vi "Bind Timestamp (Text).vi"(8 "error in (no error)":errorcluster, 10 "Time Stamp":timestamp, 11 "SQL Statement in":refnum<class "SQL Statement.lvclass">) -> (0 "error out":errorcluster, 3 "SQL Statement out":refnum<class "SQL Statement.lvclass">)   [LabVIEW 2011, in "SQLite.lvlib" / "SQL Statement.lvclass"]
doc: "Bind a Timestamp as TEXT in ISO8601 format:\n\nYYYY-MM-DDTHH:MM:SS.SSSZ"
uses:
  SQL Statement.lvclass
  SQL Statement.lvclass/SQL Statement.ctl
  Error Message.vi
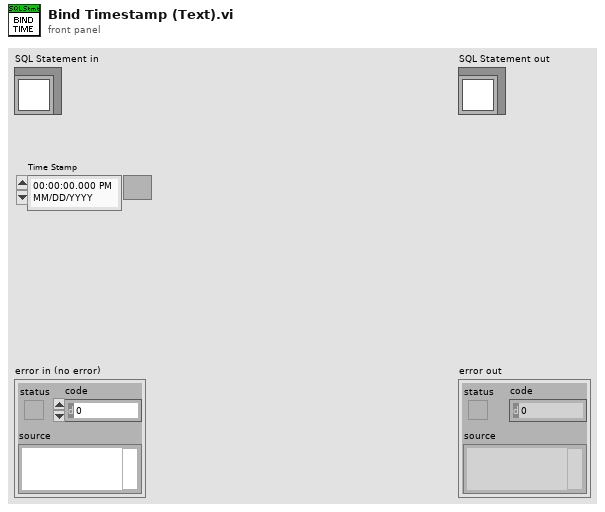
[diagram p1: front panel]
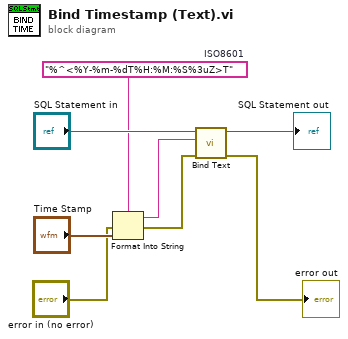
[diagram p0: block diagram]
diagram:
  w4 = "%^<%Y-%m-%dT%H:%M:%S%3uZ>T"  # ISO8601
  n1 = Format Into String(format string=w4, error in="error in (no error)", "Time Stamp") -> (resulting string=w3:string, error out=w1:errorcluster)  [unwired: 1 in]
  n2 = call "Bind Text.vi"("error in (no error)"=w1, "Text"=w3, "SQL Statement in"="SQL Statement in") -> ("error out"=→"error out":errorcluster, "SQL Statement out"=→"SQL Statement out":refnum<class "SQL Statement.lvclass">)  [unwired: 7 in]
